vi "Anti-Spam Tester.vi"() -> ()   [LabVIEW 2016, in "Anti-Spam Tester (AST).lvlib"]
doc: "This is the Anti-Spam Tester. It tests the Anti-Spam Functionality of the Error Manager module.\n\nThe Error Manager handles* up to 5 errors of the same error code per second. If more than 5 errors of the same error code were reported in a second, the remainder errors are not handled. Nevertheless, at the end of the one-second interval, the Error Manager logs a message such as:\n\n \"Too many errors were reported in the last second. The details of the following errors were not logged:\n1. 11 instances of error 5001\n2. 25 instances of error 5002\n3. 33 instances of error 5003\"\n\n*To handle an error means to log it to the Error Log to file, and to display its details to the user using the Error Window (popup window).\n\nThe Anti-Spam Tester is important because it demonstrates the Error Manager's ability to discard spam errors. This prevents a situation where the Error Manager could become jammed by having to deal with too many errors reported in a short amount of time (e.g. 1,000 errors reported in 10 milliseconds). This can happen if the host application contains a loop that iterates quickly and experiences an error on each iteration.\n\nAST = Anti-Spam Tester"
uses:
  Anti-Spam Tester (AST).lvlib
  Error Manager/Error Manager.lvlib
  MHL Queue/AST MHL Queue.lvclass
  MHL Queue/Command (enum).ctl
  GUI refs - Input (cluster).ctl
  GUI refs - Buttons (cluster).ctl
  GUI refs (cluster).ctl
  Spam Mode (enum).ctl
  Spam Frequency (enum).ctl
  Spam Error Message Type (enum).ctl
panel:
  out "Anti-Spam Tester Settings Filepath":path
  out "MHL iteration":i32
  in  "Error Message Type":T1=enum."Long Error Message"
  in  "How many error codes?":u32=3 caption="How many different error codes (different types of error)?" min=1 max=9
  in  "Spam Frequency":T2=enum."Every 10 ms"
  in  "Stop Spamming":bool
  in  "Start Spamming":bool
  in  "n (ms)":u32=5000 min=100 max=60000 step=100
  in  "Spam Mode":T3
  out "Error Out":errorcluster
  in  "Include call chain?":bool=TRUE
  in  "Show Error Manager GUI":bool
  in  "Exit Tester":bool
  out "EHL iteration":i32
  # "Anti-Spam Tester\nThis VI tests the Anti-Spam Functionality of the Error Manager module."
  # "Input"
  # "Control"
  # "Output"
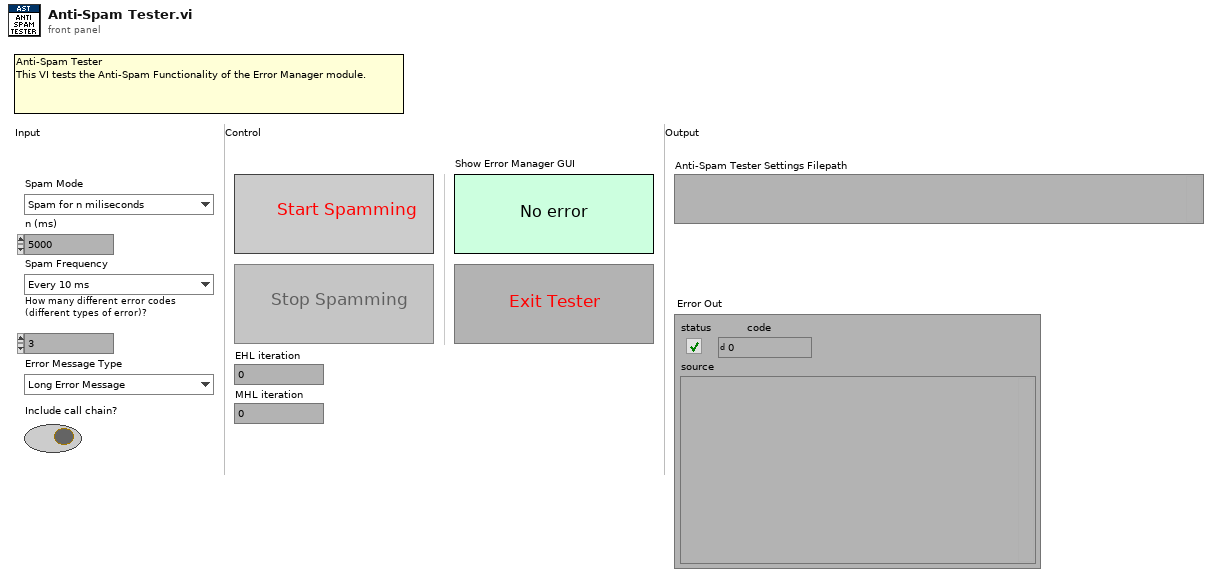
[diagram p1: front panel]
types:
  T1 = typedef "Anti-Spam Tester (AST).lvlib/Spam Error Message Type (enum).ctl" = enum16{"Short Error Message", "Long Error Message"}
  T2 = typedef "Anti-Spam Tester (AST).lvlib/Spam Frequency (enum).ctl" = enum16{"As fast as possible", "Every 1 ms", "Every 2 ms", "Every 5 ms", "Every 10 ms", "Every 20 ms", "Every 50 ms", "Every 100 ms", "Every 200 ms", "Every 500 ms", "Every 1000 ms"}
  T3 = typedef "Anti-Spam Tester (AST).lvlib/Spam Mode (enum).ctl" = enum16{"Spam for n miliseconds", "Spam continuously"}
  T4 = typedef "Anti-Spam Tester (AST).lvlib/AST MHL Queue.lvclass/Command (enum).ctl" = enum16{"Init AST", "Close AST", "Config GUI - Init", "Config GUI - Spamming Has Started", "Config GUI - Spamming Has Stopped", "Spam"}
  T5 = typedef "Anti-Spam Tester (AST).lvlib/GUI refs - Buttons (cluster).ctl" = cluster{"Start Spamming":refnum<vi>, "Stop Spamming":refnum<vi>}
  T6 = typedef "Anti-Spam Tester (AST).lvlib/GUI refs - Input (cluster).ctl" = cluster{"Spam Mode":refnum<vi>, "n (ms)":refnum<vi>, "Spam Frequency":refnum<vi>, "How many error codes?":refnum<vi>, "Spam Error Message Type":refnum<vi>, "Include call chain?":refnum<vi>}
  T7 = typedef "Anti-Spam Tester (AST).lvlib/GUI refs (cluster).ctl" = cluster{"Input":T6, "Buttons":T5}
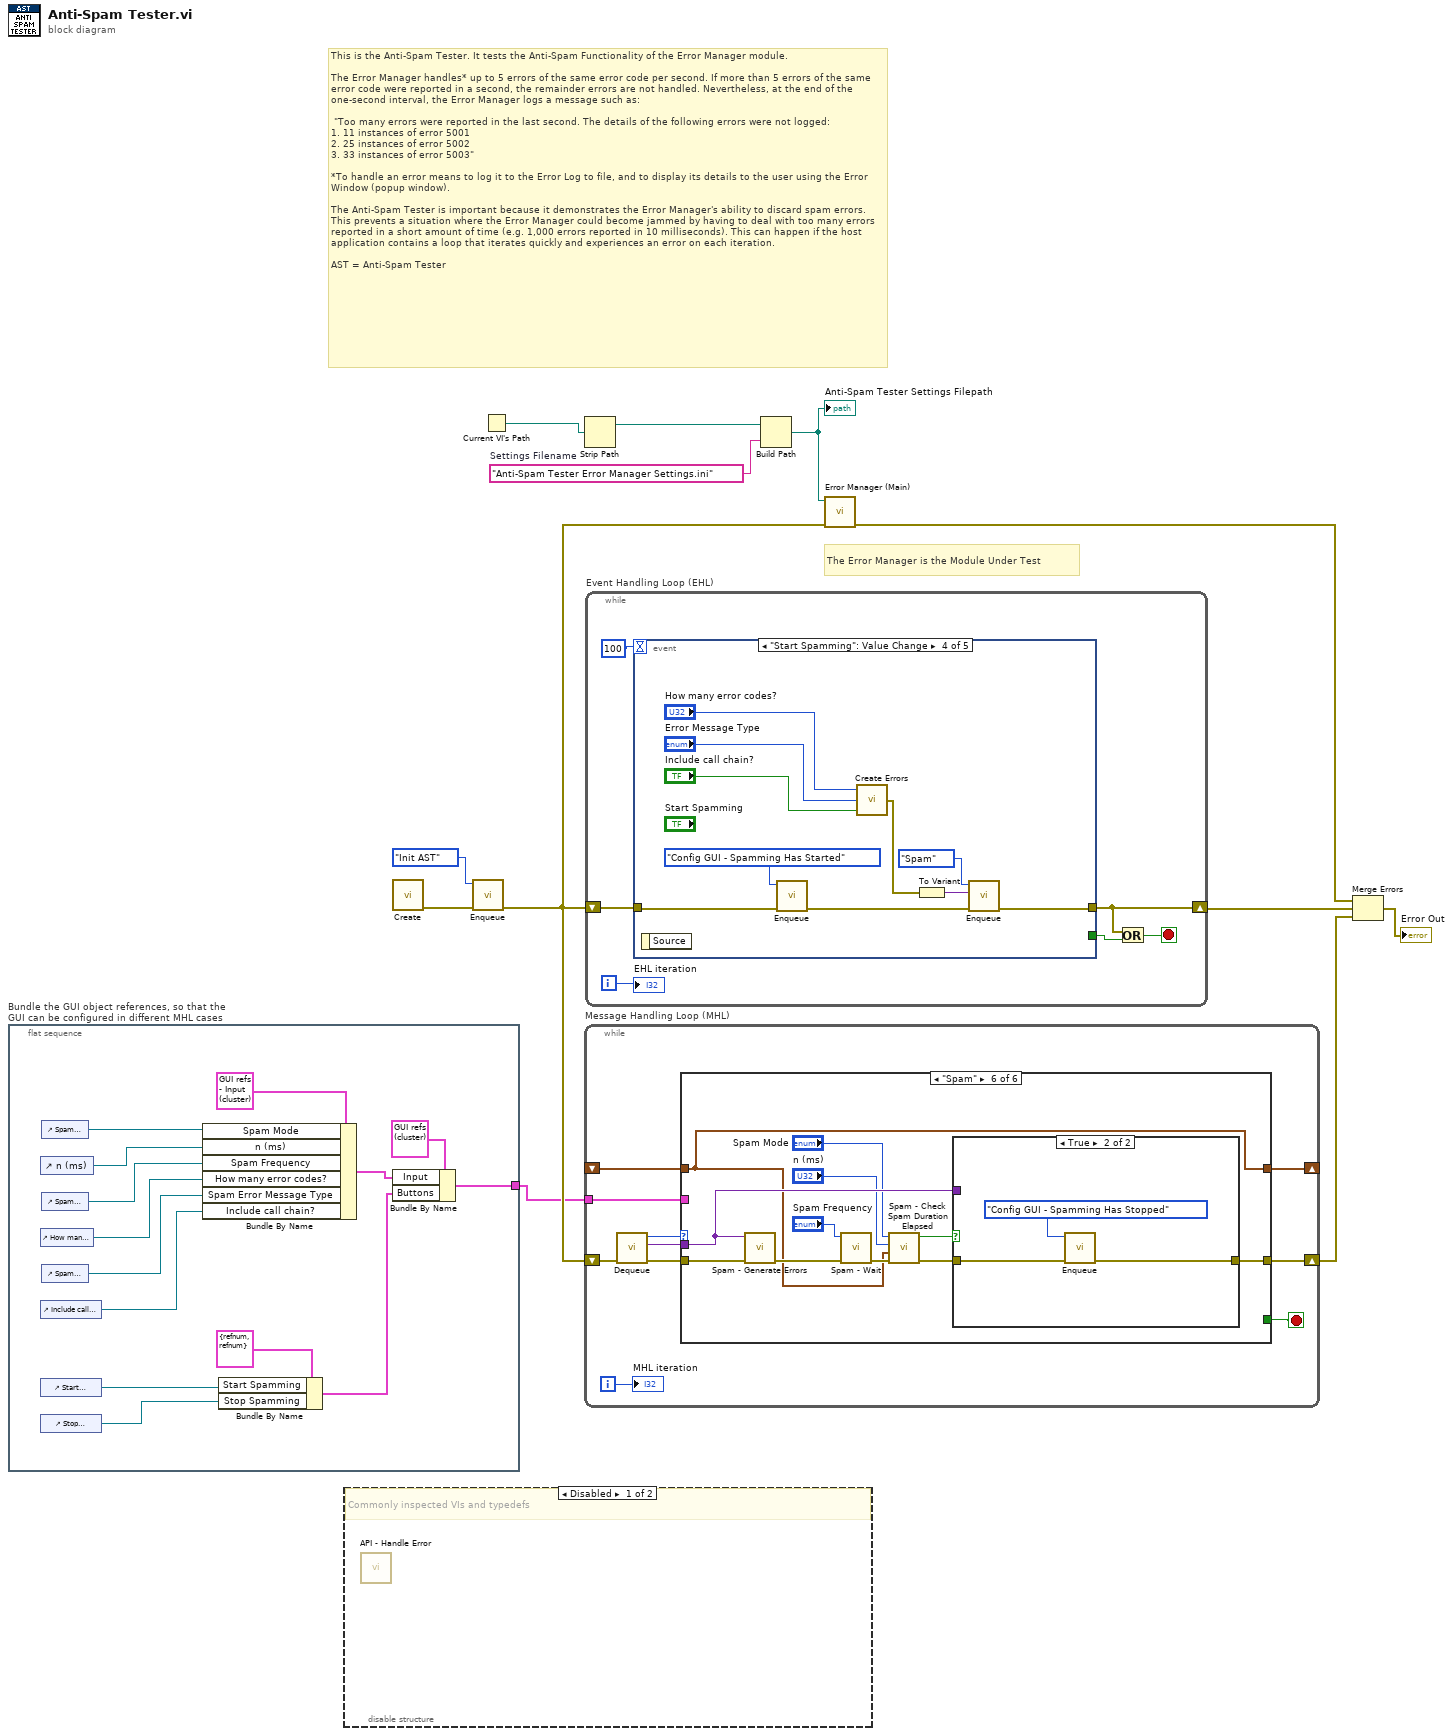
[diagram p0: block diagram]
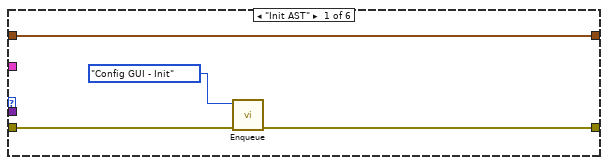
[diagram p3: hidden frame]
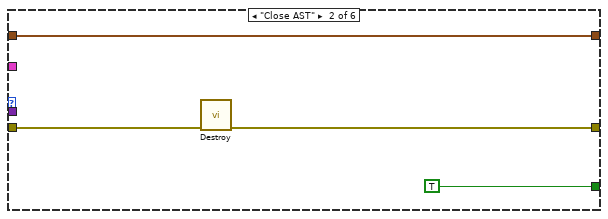
[diagram p4: hidden frame]
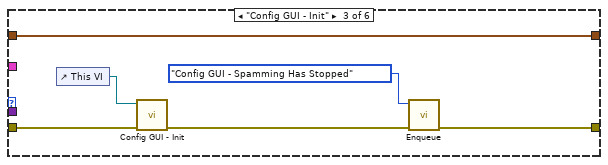
[diagram p5: hidden frame]
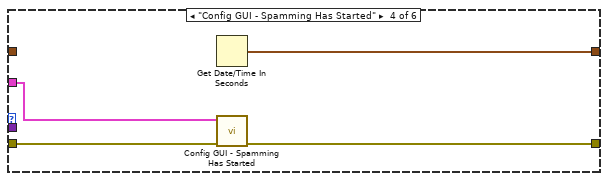
[diagram p6: hidden frame]
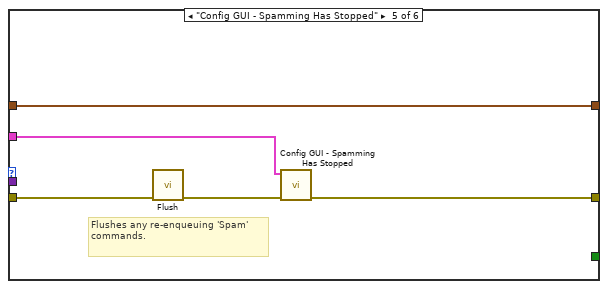
[diagram p7: hidden frame]
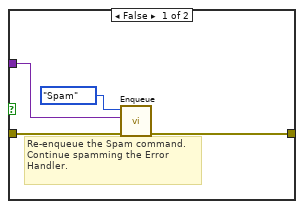
[diagram p8: hidden frame]
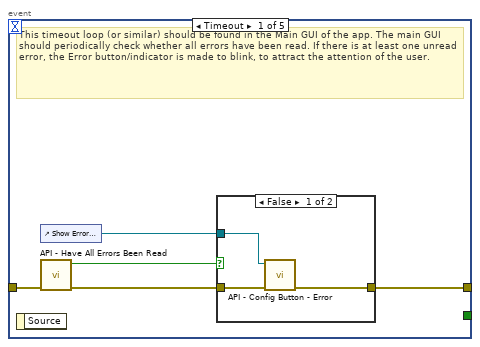
[diagram p9: hidden frame]
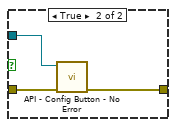
[diagram p10: hidden frame]
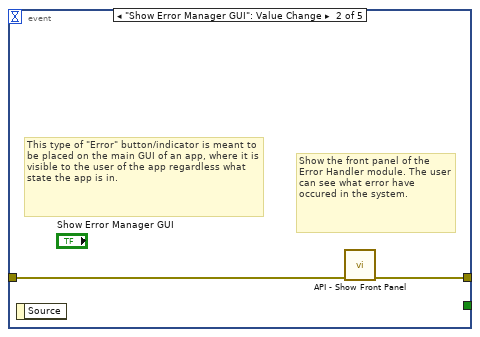
[diagram p11: hidden frame]
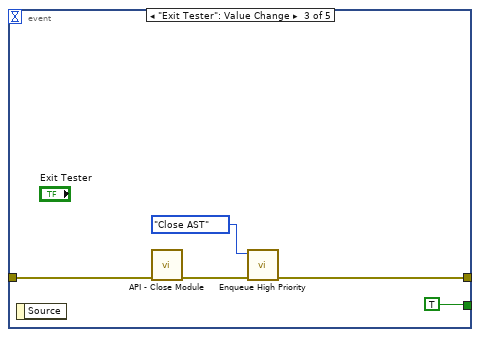
[diagram p12: hidden frame]
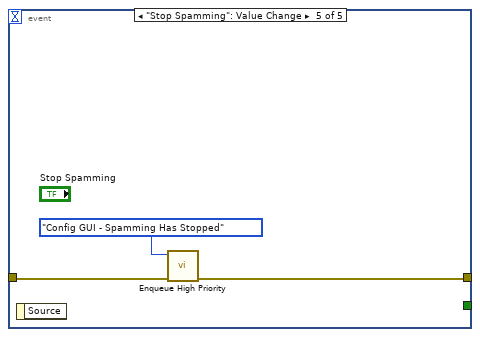
[diagram p13: hidden frame]
diagram:
  w2 = "Anti-Spam Tester Error Manager Settings.ini"  # Settings Filename
  # "The Error Manager is the Module Under Test"
  # "This is the Anti-Spam Tester. It tests the Anti-Spam Functionality of the Error Manager module.\n\nThe Error Manager handles* up to 5 errors of the same error code per second. If more than 5 errors of the same error code were reported in a second, the remainder errors are not handled. Nevertheless, at the end of the one-second interval, the Error Manager logs a message such as:\n\n \"Too many errors were reported in the last second. The details of the following errors were not logged:\n1. 11 instances of error 5001\n2. 25 instances of error 5002\n3. 33 instances of error 5003\"\n\n*To handle an error means to log it to the Error Log to file, and to display its details to the user using the Error Window (popup window).\n\nThe Anti-Spam Tester is important because it demonstrates the Error Manager's ability to discard spam errors. This prevents a situation where the Error Manager could become jammed by having to deal with too many errors reported in a short amount of time (e.g. 1,000 errors reported in 10 milliseconds). This can happen if the host application contains a loop that iterates quickly and experiences an error on each iteration.\n\nAST = Anti-Spam Tester"
  n1 = flat-sequence "Bundle the GUI object references, so that the GUI can be configured in different MHL cases" {
    tunnel: [w13] -> w5
    frame #0 {
      n2 = control-ref of="n (ms)"() -> (w18:refnum<vi>)
      n3 = control-ref of="How many error codes?"() -> (w16:refnum<vi>)
      n4 = control-ref of="Include call chain?"() -> (w14:refnum<vi>)
      n5 = control-ref of="Start Spamming"() -> (w21:refnum<vi>)
      n6 = control-ref of="Stop Spamming"() -> (w20:refnum<vi>)
      n7 = control-ref of="Spam Mode"() -> (w19:refnum<vi>)
      n8 = control-ref of="Spam Frequency"() -> (w17:refnum<vi>)
      n9 = control-ref of="Spam Error Message Type"() -> (w15:refnum<vi>)
      n10 = Bundle By Name(cluster=T6 {"Spam Mode"=refnum, "n (ms)"=refnum, "Spam Frequency"=refnum, "How many error codes?"=refnum, "Spam Error Message Type"=refnum, "Include call chain?"=refnum} ("GUI refs - Input"), "Spam Mode"=w19, "n (ms)"=w18, "Spam Frequency"=w17, "How many error codes?"=w16, "Spam Error Message Type"=w15, "Include call chain?"=w14) -> (w24:T6)
      n11 = Bundle By Name(cluster=T5 {"Start Spamming"=refnum, "Stop Spamming"=refnum} ("GUI refs - Buttons"), "Start Spamming"=w21, "Stop Spamming"=w20) -> (w22:T5)
      n12 = Bundle By Name(cluster=T7 {"Input"={"Spam Mode"=refnum, "n (ms)"=refnum, "Spam Frequency"=refnum, "How many error codes?"=refnum, "Spam Error Message Type"=refnum, "Include call chain?"=refnum}, "Buttons"={"Start Spamming"=refnum, "Stop Spamming"=refnum}} ("GUI refs"), "Input"=w24, "Buttons"=w22) -> (w13:T7)
    }
  }
  n13 = disable-structure shown="Disabled" {
    frame Disabled {
      # "Commonly inspected VIs and typedefs"
      n14 = call "API - Handle Error.vi"() -> ()  [unwired: 11 in, 1 out]
    }
    frame Enabled {
    }
  }
  n15 = call "Create.vi"() -> ("error out"=w9:errorcluster)  [unwired: 11 in]
  n16 = call "Enqueue.vi"("error in (no error)"=w9, "Command"=Command_(enum)."Init AST") -> ("error out"=w7:errorcluster)  [unwired: 9 in]
  n17 = Current VI's Path() -> (path=w4:path)
  n18 = Strip Path(path=w4) -> (stripped path=w3:path)  [unwired: 1 out]
  n19 = while "Message Handling Loop (MHL)" {
    shift-right: [w33] -> w6
    shift-left: w7 -> [w36]
    tunnel: w5 -> [w30]
    shift-right: [w28] -> _
    shift-left: _ -> [w27]
    i -> [w31]
    stop <- w32 stop-if-true
    n20 = call "Dequeue.vi"("error in (no error)"=w36) -> ("error out"=w35:errorcluster, "Data"=w29:variant, "Command"=w34:T4)  [unwired: 8 in]
    n21 = case shown="\"Spam\"" w34 {
      tunnel: w35 -> [w39 w44 w47 w54 w59 w70]
      tunnel: [w38 w43 w48 w53 w58 w65] -> w33
      tunnel: [_ TRUE _ _ _ _] -> w32
      tunnel: w30 -> [_ _ _ w52 w57 _]
      tunnel: w29 -> [_ _ _ _ _ w64]
      tunnel: [w37 w41 w45 w51 w55 w61] -> w28
      tunnel: w27 -> [w37 w41 w45 _ w55 w61]
      frame "Init AST" {
        n22 = call "Enqueue.vi"("error in (no error)"=w39, "Command"=Command_(enum)."Config GUI - Init") -> ("error out"=w38:errorcluster)  [unwired: 9 in]
      }
      frame "Close AST" {
        n23 = call "Destroy.vi"("error in (no error)"=w44) -> ("error out"=w43:errorcluster)  [unwired: 8 in, 2 out]
      }
      frame "Config GUI - Init" {
        n24 = control-ref of="This VI"() -> (w46:refnum<vi>)
        n25 = call "Config GUI - Init.vi"("error in (no error)"=w47, "VI Reference"=w46) -> ("error out"=w49:errorcluster)  [unwired: 9 in]
        n26 = call "Enqueue.vi"("error in (no error)"=w49, "Command"=Command_(enum)."Config GUI - Spamming Has Stopped") -> ("error out"=w48:errorcluster)  [unwired: 9 in]
      }
      frame "Config GUI - Spamming Has Started" {
        n27 = Get Date/Time In Seconds() -> (seconds since 1Jan1904=w51:timestamp)
        n28 = call "Config GUI - Spamming Has Started.vi"("error in (no error)"=w54, "GUI refs"=w52) -> ("error out"=w53:errorcluster)  [unwired: 9 in]
      }
      frame "Config GUI - Spamming Has Stopped" {
        # "Flushes any re-enqueuing 'Spam' commands."
        n29 = call "Flush.vi"("error in (no error)"=w59) -> ("error out"=w56:errorcluster)  [unwired: 8 in, 2 out]
        n30 = call "Config GUI - Spamming Has Stopped.vi"("error in (no error)"=w56, "GUI refs"=w57) -> ("error out"=w58:errorcluster)  [unwired: 9 in]
      }
      frame "Spam" {
        n31 = call "Spam - Generate Errors.vi"("error in (no error)"=w70, "Variant"=w64) -> ("error out"=w67:errorcluster)  [unwired: 9 in]
        n32 = call "Spam - Wait.vi"("error in (no error)"=w67, "Spam Frequency"="Spam Frequency") -> ("error out"=w68:errorcluster)  [unwired: 9 in]
        n33 = call "Spam - Check Spam Duration Elapsed.vi"("error in (no error)"=w68, "Spam Started Timestamp"=w61, "n (ms)"="n (ms)", "Spam Mode"="Spam Mode") -> ("error out"=w66:errorcluster, "T = Spam duration has elapsed. Need to stop spamming."=w60:bool)  [unwired: 6 in]
        n34 = case shown="True" w60 {
          tunnel: w66 -> [w73 w76]
          tunnel: [w72 w75] -> w65
          tunnel: w64 -> [w71 _]
          frame False {
            # "Re-enqueue the Spam command. Continue spamming the Error Handler."
            n35 = call "Enqueue.vi"("error in (no error)"=w73, "Data"=w71, "Command"=Command_(enum)."Spam") -> ("error out"=w72:errorcluster)  [unwired: 8 in]
          }
          frame True {
            n36 = call "Enqueue.vi"("error in (no error)"=w76, "Command"=Command_(enum)."Config GUI - Spamming Has Stopped") -> ("error out"=w75:errorcluster)  [unwired: 9 in]
          }
        }
      }
    }
    "MHL iteration" <- w31
  }
  n37 = while "Event Handling Loop (EHL)" {
    shift-right: [w80] -> w11
    shift-left: w7 -> [w81]
    i -> [w83]
    stop <- w78 stop-if-true
    n38 = event shown="[3] \"Start Spamming\": Value Change" {
      selector: _ -> [_ _ _ _ _]
      dyn-events: _ -> [_ _ _ _ _]
      timeout: 100 -> [_ _ _ _ _]
      tunnel: w81 -> [w88 w96 w100 w110 w113]
      tunnel: [w86 w95 w98 w107 w112] -> w80
      tunnel: [_ _ TRUE _ _] -> w79
      event Timeout {
        # "This timeout loop (or similar) should be found in the Main GUI of the app. The main GUI should periodically check whether all errors have been read. If there is at least one unread error, the Error button/indicator is made to blink, to attract the attention of the user."
        n39 = event-data() -> ()  [unwired: 1 in, 1 out]
        n40 = control-ref of="Show Error Manager GUI"() -> (w84:refnum<vi>)
        n41 = call "API - Have All Errors Been Read.vi"("error in"=w88) -> ("error out"=w87:errorcluster, "Have All Errors Been Read?"=w85:bool)  [unwired: 9 in]
        n42 = case shown="False" w85 {
          tunnel: [w89 w93] -> w86
          tunnel: w87 -> [w90 w94]
          tunnel: w84 -> [w91 w92]
          frame False {
            n43 = call "API - Config Button - Error.vi"("error in"=w90, "Error Button"=w91) -> ("error out"=w89:errorcluster)  [unwired: 9 in]
          }
          frame True {
            n44 = call "API - Config Button - No Error.vi"("error in"=w94, "Error Button"=w92) -> ("error out"=w93:errorcluster)  [unwired: 9 in]
          }
        }
      }
      event "Show Error Manager GUI": Value Change {
        # "This type of \"Error\" button/indicator is meant to be placed on the main GUI of an app, where it is visible to the user of the app regardless what state the app is in."
        # "Show the front panel of the Error Handler module. The user can see what error have occured in the system."
        n45 = event-data() -> ()  [unwired: 1 in, 1 out]
        n46 = call "API - Show Front Panel.vi"("error in"=w96) -> ("error out"=w95:errorcluster)  [unwired: 10 in]
      }
      event "Exit Tester": Value Change {
        n47 = event-data() -> ()  [unwired: 1 in, 1 out]
        n48 = call "API - Close Module.vi"("error in"=w100) -> ("error out"=w101:errorcluster)  [unwired: 10 in]
        n49 = call "Enqueue High Priority.vi"("error in (no error)"=w101, "Command"=Command_(enum)."Close AST") -> ("error out"=w98:errorcluster)  [unwired: 9 in]
      }
      event "Start Spamming": Value Change {
        n50 = event-data() -> ()  [unwired: 1 in, 1 out]
        n51 = call "Enqueue.vi"("error in (no error)"=w110, "Command"=Command_(enum)."Config GUI - Spamming Has Started") -> ("error out"=w108:errorcluster)  [unwired: 9 in]
        n52 = call "Create Errors.vi"("Show call chain?"="Include call chain?", "Error Message Type"="Error Message Type", "Number of different error codes"="How many error codes?") -> ("Errors"=w106:errorcluster[])
        n53 = To Variant(anything=w106) -> (Variant=w105:variant)
        n54 = call "Enqueue.vi"("error in (no error)"=w108, "Data"=w105, "Command"=Command_(enum)."Spam") -> ("error out"=w107:errorcluster)  [unwired: 8 in]
      }
      event "Stop Spamming": Value Change {
        n55 = event-data() -> ()  [unwired: 1 in, 1 out]
        n56 = call "Enqueue High Priority.vi"("error in (no error)"=w113, "Command"=Command_(enum)."Config GUI - Spamming Has Stopped") -> ("error out"=w112:errorcluster)  [unwired: 9 in]
      }
    }
    n57 = Or(x=w80, y=w79) -> (x .or. y?=w78:bool)
    "EHL iteration" <- w83
  }
  n58 = Build Path(base path=w3, name or relative path=w2) -> (appended path=w1:path)
  "Anti-Spam Tester Settings Filepath" <- w1
  n59 = call "Error Manager (Main).vi"("Error In"=w7, "Settings Filepath"=w1) -> ("Error Out"=w12:errorcluster)  [unwired: 9 in]
  n60 = Merge Errors(w12, w11, w6) -> (→"Error Out":errorcluster)
